vi "subFindProjects.vi"(8 "error in (no error)":errorcluster, 11 "SolutionBuilder in":refnum<class "SolutionBuilder.lvclass">) -> (0 "error out":errorcluster, 3 "SolutionBuilder out":refnum<class "SolutionBuilder.lvclass">)   [LabVIEW 2019, in "SolutionBuilder.lvlib" / "SolutionBuilder.lvclass"]
uses:
  SolutionBuilder.lvclass
  SolutionBuilder.lvclass/SolutionBuilder.ctl
  ProjectItem/ProjectItem.lvclass
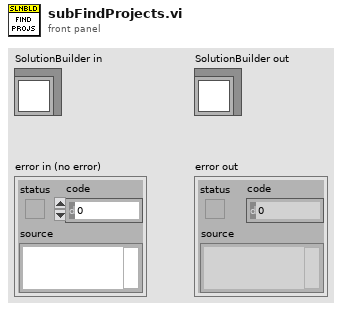
[diagram p1: front panel]
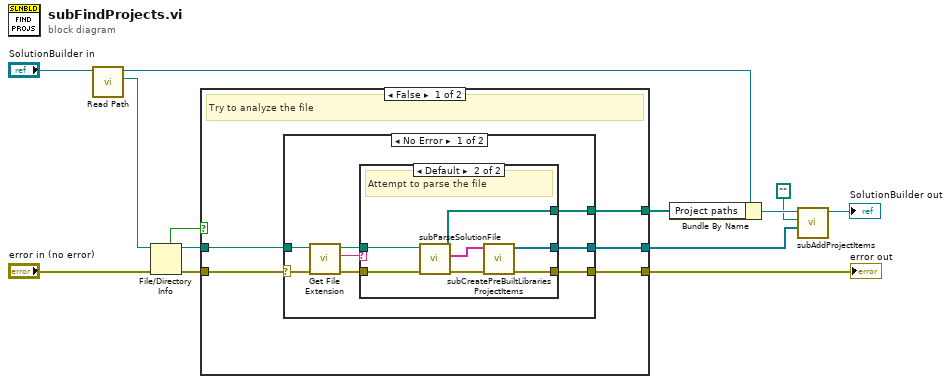
[diagram p0: block diagram]
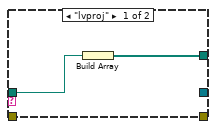
[diagram p2: hidden frame]
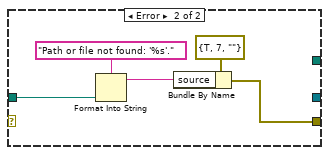
[diagram p3: hidden frame]
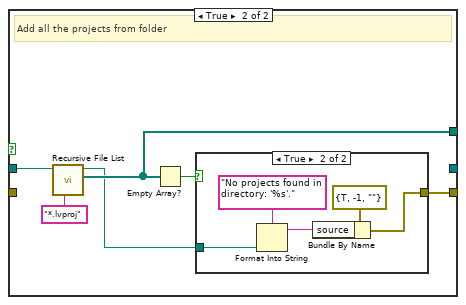
[diagram p4: hidden frame]
diagram:
  n1 = call-dynamic "Read Path.vi"("SolutionBuilder in"="SolutionBuilder in") -> ("Path"=w9:path, "SolutionBuilder out"=w8:refnum<class "SolutionBuilder.lvclass">)  [unwired: 9 in]
  n2 = File/Directory Info(path=w9, error in="error in (no error)") -> (path out=w12:path, directory=w13:bool, error out=w11:errorcluster)  [unwired: 4 out]
  n3 = case shown="False" w13 {
    tunnel: [w16 w44] -> w5
    tunnel: w12 -> [w18 w43]
    tunnel: w11 -> [w17 _]
    tunnel: [w15 w45] -> w6
    tunnel: [w14 _] -> w1
    frame False {
      # "Try to analyze the file"
      n4 = case shown="No Error" w17 {
        selector: w17 -> [w25 _]
        tunnel: w18 -> [w24 w38]
        tunnel: [w26 _] -> w16
        tunnel: [w20 w37] -> w15
        tunnel: [w19 _] -> w14
        frame No Error {
          n5 = call <vilib>:"Get File Extension.vi"("error in (no error)"=w25, "file"=w24) -> ("error out"=w22:errorcluster, "lowercase file extension"=w21:string, "dup file"=w23:path)  [unwired: 5 in, 2 out]
          n6 = case shown="Default" w21 {
            tunnel: [w27 w35] -> w26
            tunnel: w23 -> [w28 w33]
            tunnel: w22 -> [_ w34]
            tunnel: [_ w30] -> w20
            tunnel: [_ w29] -> w19
            frame "lvproj" {
              n7 = Build Array(w28) -> (w27:path[])
            }
            frame Default {
              # "Attempt to parse the file"
              n8 = call "subParseSolutionFile.vi"("error in (no error)"=w34, "Solution file"=w33) -> ("error out"=w31:errorcluster, "Lib definition strings"=w32:string[], "Projects"=w35:path[])  [unwired: 7 in]
              n9 = call "subCreatePreBuiltLibrariesProjectItems.vi"("error in"=w31, "Lib definition strings"=w32) -> ("error out"=w30:errorcluster, "Pre-built libraries"=w29:refnum<class "ProjectItem.lvclass">[])  [unwired: 8 in]
            }
          }
        }
        frame Error {
          n10 = Format Into String(format string="Path or file not found: '%s'.", w38) -> (resulting string=w39:string)  [unwired: 2 in, 1 out]
          n11 = Bundle By Name(cluster=errorcluster {"status"=TRUE, "code"=7, "source"=""} ("t"), "source"=w39) -> (w37:errorcluster)
        }
      }
    }
    frame True {
      # "Add all the projects from folder"
      n12 = call <vilib>:"Recursive File List.vi"("pattern"="*.lvproj", "Folder Path"=w43) -> ("All Files in Dir"=w44:path[], "dup Folder Path"=w42:path)  [unwired: 5 in, 3 out]
      n13 = Empty Array?(array=w44) -> (empty?=w41:bool)
      n14 = case shown="True" w41 {
        tunnel: [_ w48] -> w45
        tunnel: w42 -> [_ w47]
        frame False {
        }
        frame True {
          n15 = Format Into String(format string="No projects found in directory: '%s'.", w47) -> (resulting string=w50:string)  [unwired: 2 in, 1 out]
          n16 = Bundle By Name(cluster=errorcluster {"status"=TRUE, "code"=-1, "source"=""} ("t"), "source"=w50) -> (w48:errorcluster)
        }
      }
    }
  }
  "error out" <- w6
  n17 = Bundle By Name(cluster=w8, "Project paths"=w5) -> (w4:refnum<class "SolutionBuilder.lvclass">)
  n18 = call "subAddProjectItems.vi"("ProjectItems"=w1, "Owning project"=path "", "SolutionBuilder in"=w4) -> ("SolutionBuilder out"=→"SolutionBuilder out":refnum<class "SolutionBuilder.lvclass">)  [unwired: 7 in, 1 out]
